vi "Tree2Array.vi"(11 "TreeControl输入":refnum<vi>) -> (2 "循环数组":string[](array[string]), 3 "TreeControl输出":refnum<vi>)   [LabVIEW 2020, in "Curve Editor.lvlib"]
uses:
  Curve Editor.lvlib
panel:
  # "将树形列表转换为字符串数组"
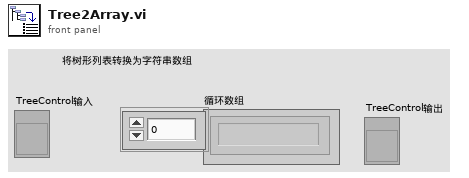
[diagram p1: front panel]
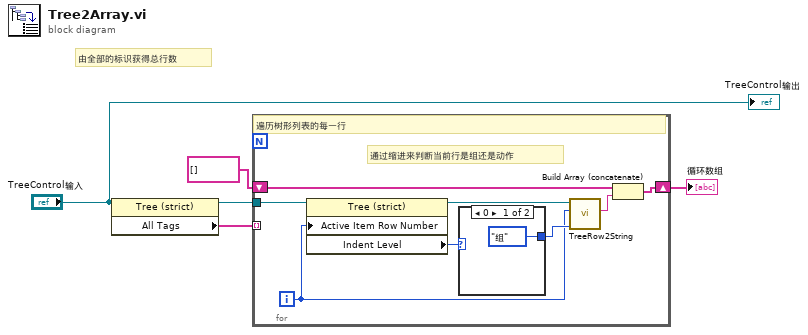
[diagram p0: block diagram]
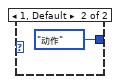
[diagram p2: hidden frame]
diagram:
  # "由全部的标识获得总行数"
  n1 = property class="Tree (strict)"(reference="TreeControl输入") -> (reference out=w4:refnum<vi>, "All Tags"=w3:string[])  [unwired: 1 in, 1 out]
  n2 = for {
    tunnel: w3 -> [_] mode=indexing
    tunnel: w4 -> [w13]
    shift-right: [w7] -> w2
    shift-left: string[] [] -> [w8]
    i -> [w9]
    # "通过缩进来判断当前行是组还是动作"
    # "遍历树形列表的每一行"
    n3 = property class="Tree (strict)"(reference=w13, "Active Item Row Number"=w9) -> (reference out=w10:refnum<vi>, "Indent Level"=w12:i32)  [unwired: 1 in, 1 out]
    n4 = case shown="0" w12 {
      tunnel: [enum16{"动作", "组"}."组" ("类型") enum16{"动作", "组"}."动作" ("类型")] -> w11
      frame 0 {
      }
      frame 1, Default {
      }
    }
    n5 = call "TreeRow2String.vi"("类型"=w11, "索引"=w9, "TreeControl输入"=w10) -> ("键值串"=w6:string)  [unwired: 7 in, 1 out]
    n6 = Build Array (concatenate)(w8, w6) -> (w7:string[])
  }
  "循环数组" <- w2
  "TreeControl输出" <- "TreeControl输入"
